vi "CH1_Comm_TCPIP.vi"() -> ()   [LabVIEW 2018]
uses:
  RxTx/RxTx.lvclass
  TCPIP/TCPIP.lvclass
panel:
  in  "TCPIP out":refnum<class "TCPIP.lvclass">
  in  "RxTx.lvclass":refnum<class "RxTx.lvclass">
  in  "Channel:":u16=1
  out "error out 4":errorcluster
  out "error out 2":errorcluster
  out "error out":errorcluster
  in  "IP":string="200.131.64.49"
  in  "remote port":u16=59041
  in  "error out 3":errorcluster
  in  "stop":bool
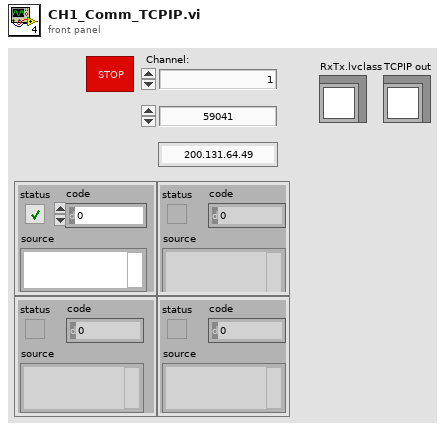
[diagram p1: front panel]
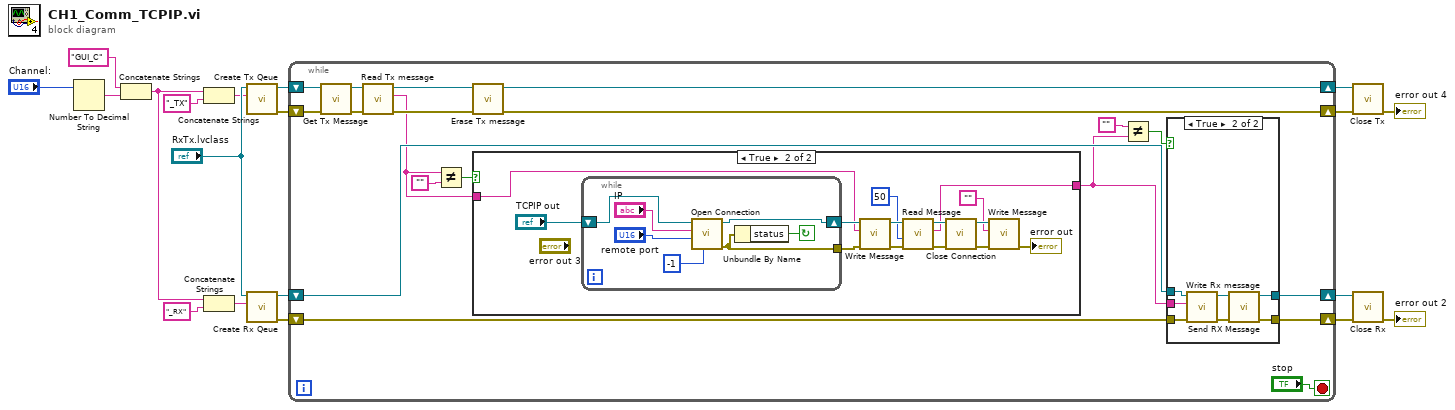
[diagram p0: block diagram]
diagram:
  n1 = Number To Decimal String(number="Channel:") -> (decimal integer string=w19:string)  [unwired: 1 in]
  n2 = Concatenate Strings("GUI_C", w19) -> (w14:string)
  n3 = Concatenate Strings(w14, "_TX" ("Reader Name")) -> (w1:string)
  n4 = Concatenate Strings(w14, "_RX" ("Reader Name")) -> (w2:string)
  n5 = call "Create Tx Qeue.vi"("Writer Name"=w1, "RxTx in"="RxTx.lvclass") -> ("error out"=w10:errorcluster, "RxTx out"=w11:refnum<class "RxTx.lvclass">)  [unwired: 8 in]
  n6 = call "Create Rx Qeue.vi"("Reader Name"=w2, "RxTx in"="RxTx.lvclass") -> ("error out"=w12:errorcluster, "RxTx out"=w13:refnum<class "RxTx.lvclass">)  [unwired: 8 in]
  n7 = while {
    shift-right: [w26] -> w8
    shift-left: w10 -> [w28]
    shift-right: [w27] -> w9
    shift-left: w11 -> [w29]
    shift-right: [w34] -> w7
    shift-left: w13 -> [w35]
    shift-right: [w33] -> w6
    shift-left: w12 -> [w36]
    stop <- "stop" stop-if-true
    n8 = call "Get Tx Message.vi"("error in (no error)"=w28, "RxTx in"=w29) -> ("error out"=w24:errorcluster, "RxTx out"=w25:refnum<class "RxTx.lvclass">)  [unwired: 8 in]
    n9 = call "Read Tx message.vi"("error in (no error)"=w24, "RxTx in"=w25) -> ("error out"=w23:errorcluster, "Tx Message"=w21:string, "RxTx out"=w22:refnum<class "RxTx.lvclass">)  [unwired: 7 in]
    n10 = Not Equal?(x=w21, y="") -> (x != y?=w37:bool)
    n11 = call "Erase Tx message.vi"("error in (no error)"=w23, "RxTx in"=w22) -> ("error out"=w26:errorcluster, "RxTx out"=w27:refnum<class "RxTx.lvclass">)  [unwired: 8 in]
    n12 = case shown="True" w37 {
      tunnel: w21 -> [_ w60]
      tunnel: [_ w54] -> w20
      frame False {
      }
      frame True {
        n13 = while {
          shift-right: [w65] -> w61
          shift-left: "TCPIP out" -> [w64]
          tunnel: [w62] -> w48
          stop <- w63 continue-if-true
          n14 = call "Open Connection.vi"("timeout"=-1, "remote port"="remote port", "IP"="IP", "TCPIP in"=w64) -> ("error out"=w62:errorcluster, "TCPIP out"=w65:refnum<class "TCPIP.lvclass">)  [unwired: 6 in]
          n15 = Unbundle By Name(w62) -> ("status"=w63:bool)
        }
        n16 = call "Write Message.vi"("error in (no error)"=w48, "Message"=w60, "TCPIP in"=w61) -> ("error out"=w58:errorcluster, "TCPIP out"=w59:refnum<class "TCPIP.lvclass">)  [unwired: 7 in]
        n17 = call "Read Message.vi"("error in (no error)"=w58, "timeout"=50, "TCPIP in"=w59) -> ("error out"=w56:errorcluster, "Message"=w54:string, "TCPIP out"=w55:refnum<class "TCPIP.lvclass">)  [unwired: 6 in]
        n18 = call "Close Connection.vi"("error in (no error)"=w56, "TCPIP in"=w55) -> ("error out"=w52:errorcluster, "TCPIP out"=w53:refnum<class "TCPIP.lvclass">)  [unwired: 8 in]
        n19 = call "Write Message.vi"("error in (no error)"=w52, "Message"="", "TCPIP in"=w53) -> ("error out"=→"error out":errorcluster)  [unwired: 7 in, 1 out]
      }
    }
    n20 = Not Equal?(x="", y=w20) -> (x != y?=w31:bool)
    n21 = case shown="True" w31 {
      tunnel: w36 -> [w39 w43]
      tunnel: w35 -> [w40 w42]
      tunnel: [w40 w46] -> w34
      tunnel: [w39 w47] -> w33
      tunnel: w20 -> [_ w41]
      frame False {
      }
      frame True {
        n22 = call "Write Rx message.vi"("error in (no error)"=w43, "Rx message"=w41, "RxTx in"=w42) -> ("error out"=w44:errorcluster, "RxTx out"=w45:refnum<class "RxTx.lvclass">)  [unwired: 7 in]
        n23 = call "Send RX Message.vi"("error in (no error)"=w44, "RxTx in"=w45) -> ("error out"=w47:errorcluster, "RxTx out"=w46:refnum<class "RxTx.lvclass">)  [unwired: 8 in]
      }
    }
  }
  n24 = call "Close Tx.vi"("error in (no error)"=w8, "RxTx in"=w9) -> ("error out"=→"error out 4":errorcluster)  [unwired: 8 in, 1 out]
  n25 = call "Close Rx.vi"("error in (no error)"=w6, "RxTx in"=w7) -> ("error out"=→"error out 2":errorcluster)  [unwired: 8 in, 1 out]
